vi "Execute.vi"(8 "error in (no error)":errorcluster, 10 "Plugin Initialize in":refnum<class "Plugin Handler Initialize.lvclass">, 11 "Plugin Handler Shifter Data Definition":T1) -> (0 "error out":errorcluster, 1 "Stop?":bool, 2 "Plugin Generic Command out":refnum<class "Plugin Handler Command.lvclass">, 3 "Plugin Handler Shifter Data Out":T1)   [LabVIEW 2011, in "Plugin Handler Initialize.lvclass"]
uses:
  Plugin Handler Initialize.lvclass
  Plugin Handler Command.lvclass
  Plugin Strict Type Definitions/Plugin Handler Shifter Data Definition.ctl
  Parent Plugin Definition/Plugin Template/Generic Plugin.lvclass
  Plugin Strict Type Definitions/Plugin Configuration Information.ctl
  User Interface/UI Command Manager/UI Command Manager.lvclass
  Plugin Load from Disk/Plugin Load from Disk.lvclass
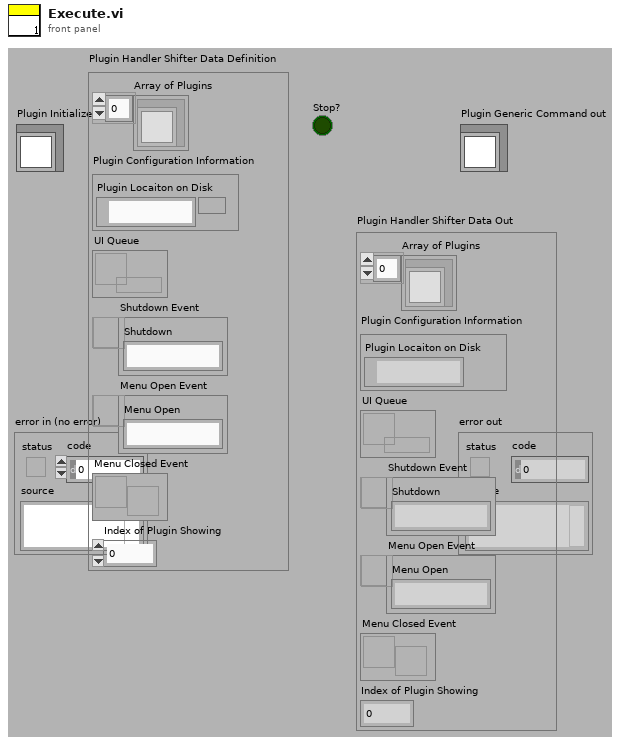
[diagram p1: front panel]
types:
  T1 = typedef "Plugin Handler Shifter Data Definition.ctl" = cluster{"Array of Plugins":refnum<class "Generic Plugin.lvclass">[], "Plugin Configuration Information":T2, "UI Queue":refnum<queue>, "Shutdown Event":refnum<user-event>, "Menu Open Event":refnum<user-event>, "Menu Closed Event":refnum<user-event>, "Index of Plugin Showing":i32}
  T2 = typedef "Plugin Configuration Information.ctl" = cluster{"Plugin Locaiton on Disk":path}
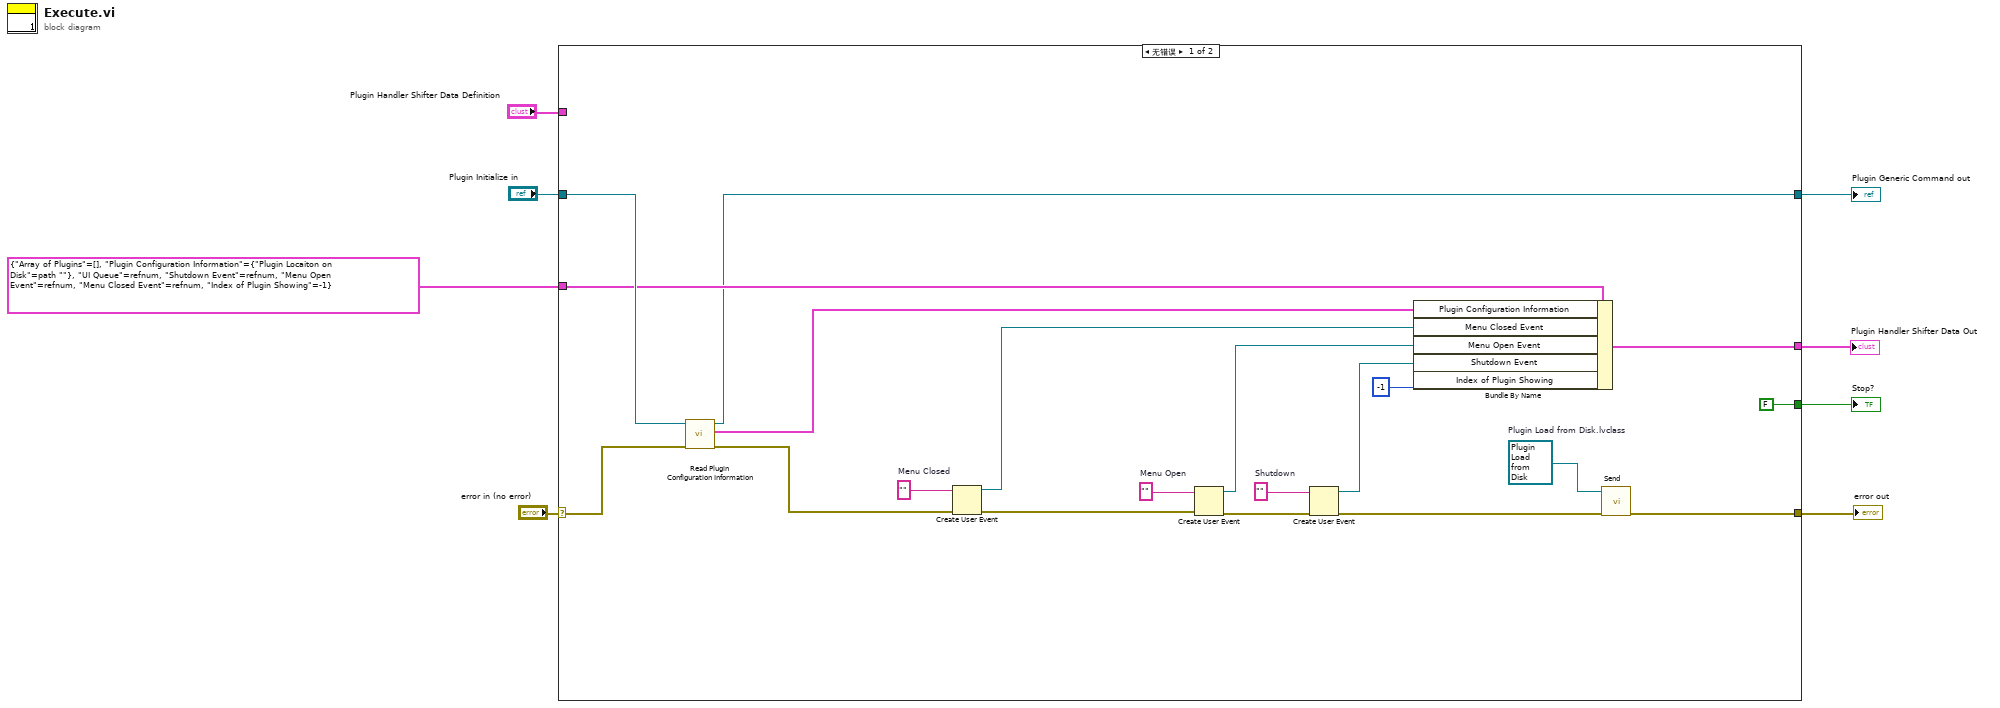
[diagram p0: block diagram]
diagram:
  n1 = case shown="无错误" "error in (no error)" {
    selector: "error in (no error)" -> [w27 w31]
    tunnel: [w20 w31] -> w1
    tunnel: [FALSE _] -> w7
    tunnel: "Plugin Initialize in" -> [w23 w30]
    tunnel: "Plugin Handler Shifter Data Definition" -> [_ _]
    tunnel: [w24 w29] -> w2
    tunnel: T1 {"Array of Plugins"=[], "Plugin Configuration Information"={"Plugin Locaiton on Disk"=path ""}, "UI Queue"=refnum, "Shutdown Event"=refnum, "Menu Open Event"=refnum, "Menu Closed Event"=refnum, "Index of Plugin Showing"=-1} ("Plugin Handler Shifter Data Definition") -> [w22 w29]
    tunnel: [w21 w30] -> w3
    frame No Error {
      w16 = ""  # Menu Closed
      w17 = ""  # Menu Open
      w19 = ""  # Shutdown
      w26 = refnum<class "Plugin Load from Disk.lvclass"> refnum  # Plugin Load from Disk.lvclass
      n2 = call "Read Plugin Configuration Information.vi"("error in (no error)"=w27, "Plugin Handler Initialize in"=w23) -> ("error out"=w13:errorcluster, "Plugin Configuration Information"=w25:T2, "Plugin Handler Initialize out"=w21:refnum<class "Plugin Handler Initialize.lvclass">)  [unwired: 7 in]
      n3 = Create User Event(user event datatype=w16, error in=w13) -> (user event=w11:refnum<user-event>, error out=w14:errorcluster)
      n4 = Create User Event(user event datatype=w17, error in=w14) -> (user event=w12:refnum<user-event>, error out=w15:errorcluster)
      n5 = Create User Event(user event datatype=w19, error in=w15) -> (user event=w10:refnum<user-event>, error out=w18:errorcluster)
      n6 = Bundle By Name(cluster=w22, "Plugin Configuration Information"=w25, "Menu Closed Event"=w11, "Menu Open Event"=w12, "Shutdown Event"=w10, "Index of Plugin Showing"=-1) -> (w24:T1)
      n7 = call "Send.vi"("error in (no error)"=w18, "Plugin Generic Command in"=w26) -> ("error out"=w20:errorcluster)  [unwired: 8 in, 1 out]
    }
    frame Error {
    }
  }
  "error out" <- w1
  "Plugin Generic Command out" <- w3
  "Stop?" <- w7
  "Plugin Handler Shifter Data Out" <- w2
